vi "EPM2000ControlLoop.vi"(8 "queue error in":errorcluster, 10 "VISA resource":refnum<visa-resource-name>, 11 "Control queue in":refnum<queue>) -> (0 "error out":errorcluster, 3 "queue out":refnum<queue>)   [LabVIEW 2013]
uses:
  EPM2K_Status.ctl
  ControlDef/MiscParams.vi
  <userlib>/Utility/ErrorLog_lib.lvlib
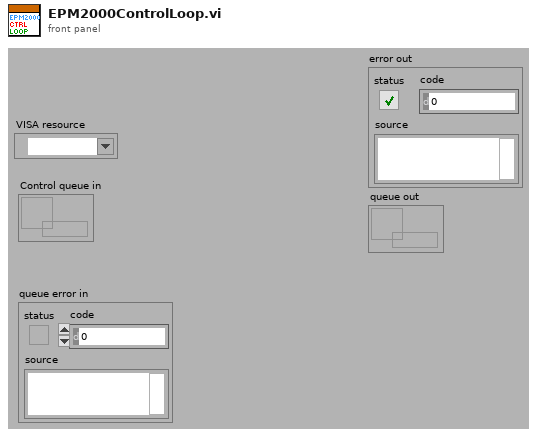
[diagram p1: front panel]
types:
  T1 = typedef "EPM2K_Status.ctl" = cluster{"State":enum16{"Initialize", "Idle/Update", "Configure", "Read", "Close", "Quit"}, "Parameter":dbl}
  T2 = enum16{"Initialize", "Write", "Write/Read", "Read", "Clear", "Close"}
  T3 = enum16{"Initialize", "Idle/Update", "Configure", "Read", "Close", "Quit"}
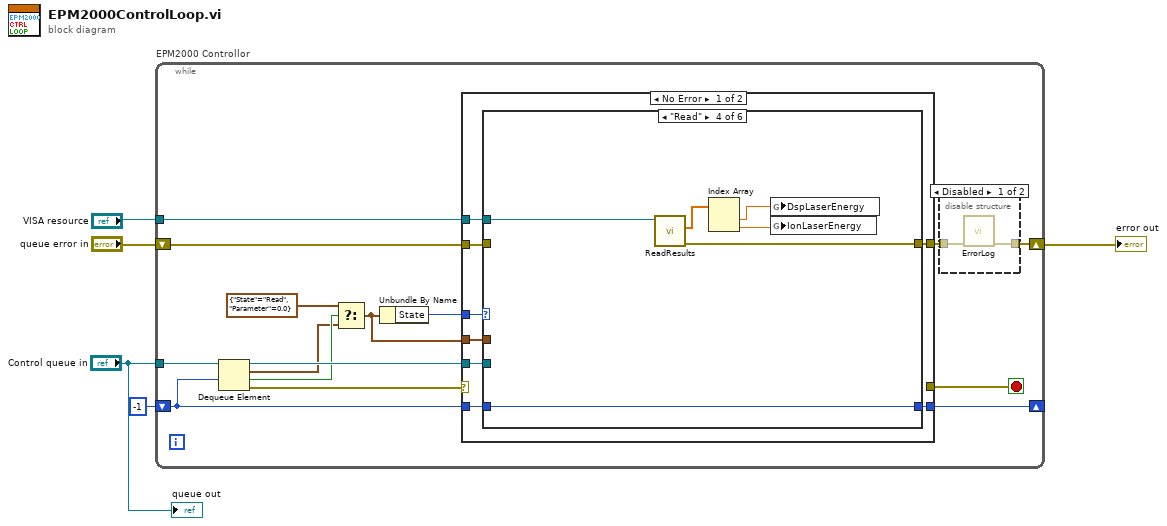
[diagram p0: block diagram]
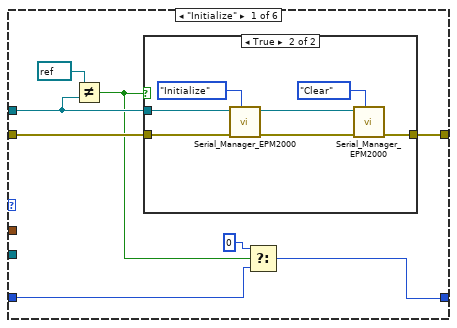
[diagram p3: hidden frame]
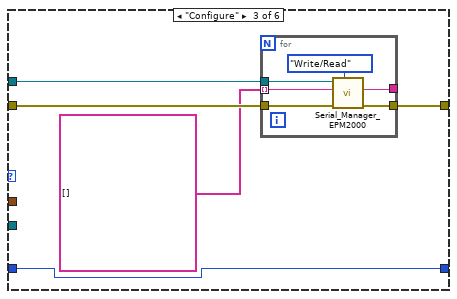
[diagram p6: hidden frame]
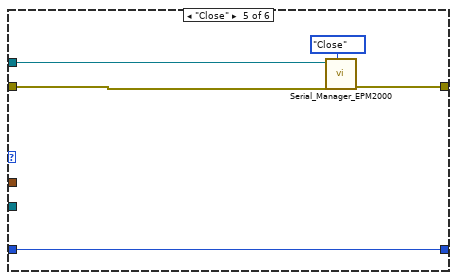
[diagram p7: hidden frame]
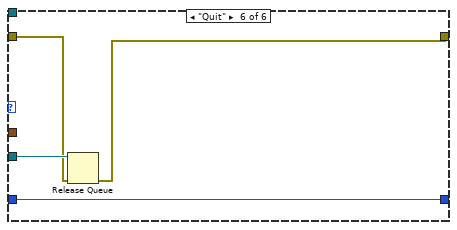
[diagram p8: hidden frame]
diagram:
  n1 = while "EPM2000 Controllor" {
    tunnel: "Control queue in" -> [w20]
    shift-right: [w8] -> w2
    shift-left: "queue error in" -> [w11]
    tunnel: "VISA resource" -> [w16]
    shift-right: [w6] -> _
    shift-left: -1 -> [w7]
    stop <- w10 stop-if-true
    n2 = Dequeue Element(queue=w20, timeout in ms (-1)=w7) -> (queue out=w19:refnum<queue>, element=w14:T1, timed out?=w17:bool, error out=w9:errorcluster)  [unwired: 1 in]
    n3 = Select(t=T1 {"State"=enum."Read", "Parameter"=0.0} ("Idle"), s=w17, f=w14) -> (s? t:f=w15:T1)
    n4 = Unbundle By Name(w15) -> ("State"=w12:T3)
    n5 = case shown="No Error" w9 {
      selector: w9 -> [_ w75]
      tunnel: w19 -> [w30 _]
      tunnel: [w29 w74] -> w18
      tunnel: w16 -> [w28 _]
      tunnel: w15 -> [w27 _]
      tunnel: w12 -> [w26 _]
      tunnel: w11 -> [w25 w74]
      tunnel: [_ w75] -> w10
      tunnel: w7 -> [w24 w73]
      tunnel: [w23 w73] -> w6
      frame No Error {
        n6 = case shown="\"Read\"" w26 {
          tunnel: w25 -> [w38 w46 w51 _ w65 w70]
          tunnel: w30 -> [_ _ _ _ _ w72]
          tunnel: w28 -> [w35 _ w49 w63 w66 _]
          tunnel: [w37 w46 w50 w62 w67 w71] -> w29
          tunnel: w27 -> [_ _ _ _ _ _]
          tunnel: w24 -> [w32 w45 w47 w58 w64 w69]
          tunnel: [w31 w45 w47 w58 w64 w69] -> w23
          frame "Initialize" {
            n7 = Not Equal?(x=refnum<visa-resource-name> refnum ("VISA resource"), y=w35) -> (x != y?=w34:bool)
            n8 = case shown="True" w34 {
              tunnel: w38 -> [_ w44]
              tunnel: [_ w40] -> w37
              tunnel: w35 -> [_ w39]
              frame False {
              }
              frame True {
                n9 = call "Serial_Manager_EPM2000.vi"("Job"=T2."Initialize", "error in"=w44, "VISA resource"=w39) -> ("error out"=w41:errorcluster)  [unwired: 7 in, 1 out]
                n10 = call "Serial_Manager_EPM2000.vi"("Job"=T2."Clear", "error in"=w41, "VISA resource"=w39) -> ("error out"=w40:errorcluster)  [unwired: 7 in, 1 out]
              }
            }
            n11 = Select(t=0, s=w34, f=w32) -> (s? t:f=w31:i32)
          }
          frame "Idle/Update" {
          }
          frame "Configure" {
            n12 = for {
              tunnel: w51 -> [w56]
              tunnel: [w55] -> w50
              tunnel: w49 -> [w54]
              tunnel: string[] [] -> [w53] mode=indexing
              tunnel: [w52] -> _
              n13 = call "Serial_Manager_EPM2000.vi"("Job"=T2."Write/Read", "error in"=w56, "write buffer"=w53, "VISA resource"=w54) -> ("error out"=w55:errorcluster, "read buffer"=w52:string)  [unwired: 6 in]
            }
          }
          frame "Read" {
            n14 = call "ReadResults.vi"("VISA resource"=w63) -> ("error out"=w62:errorcluster, "Energy/Power(SI)"=w61:dbl[])  [unwired: 9 in]
            n15 = Index Array(array=w61) -> (element #1=w60:dbl, element #2=w59:dbl)  [unwired: 2 in]
            n16 = global write "MiscParams.vi" "DspLaserEnergy"(w60) -> ()
            n17 = global write "MiscParams.vi" "IonLaserEnergy"(w59) -> ()
          }
          frame "Close" {
            n18 = call "Serial_Manager_EPM2000.vi"("Job"=T2."Close", "error in"=w65, "VISA resource"=w66) -> ("error out"=w67:errorcluster)  [unwired: 7 in, 1 out]
          }
          frame "Quit" {
            n19 = Release Queue(queue=w72, error in (no error)=w70) -> (error out=w71:errorcluster)  [unwired: 1 in, 2 out]
          }
        }
      }
      frame Error {
      }
    }
    n20 = disable-structure shown="Disabled" {
      disable-tunnel: w18 -> [w22 _]
      disable-tunnel: [w21 _] -> w8
      frame Disabled {
        n21 = call <userlib>:"ErrorLog.vi"("error in (no error)"=w22) -> ("error out"=w21:errorcluster)  [unwired: 10 in]
      }
      frame Enabled {
      }
    }
  }
  "error out" <- w2
  "queue out" <- "Control queue in"
